vi "test_Configure Response_Variable Names Error.vi"(8 "error in (no error)":errorcluster, 11 "TestCase in":refnum<class "Instrument Addon Scripting API Messages Unit Tests.lvclass">) -> (0 "error out":errorcluster, 3 "TestCase out":refnum<class "Instrument Addon Scripting API Messages Unit Tests.lvclass">)   [LabVIEW 2019, in "Instrument Addon Scripting API Messages Unit Tests.lvclass"]
uses:
  Instrument Addon Scripting API Messages Unit Tests.lvclass
  APIs/Scripting API/TypeDefs/Wait Response Settings.ctl
  APIs/Scripting API/TypeDefs/Linked Channel.ctl
  <vilib>/NI VeriStand/Custom Device API/Custom Device Item Ref.ctl
  Instrument Addon Scripting API Messages Unit Tests.lvclass/Instrument Addon Scripting API Messages Unit Tests.ctl
  Addon/Addon Shared/SubVIs/Constants.vi
  <vilib>/NI/NI VeriStand Advanced SysDef API/_SubVIs/SysDef.Search.GUID.vi
  APIs/Scripting API/Messages/Configure Response - Wait (sec).vi
  <vilib>/addons/_JKI Toolkits/VI Tester/TestCase.llb/TestCase.lvclass
  Instrument Addon Scripting API Test Assets/Instrument Addon Scripting API Test Assets.lvclass
  APIs/Scripting API/Instrument Addon Scripting API.lvlib
  <vilib>/NI VeriStand/Custom Device API/Custom Device API.lvlib
  <vilib>/NI/NI VeriStand Advanced SysDef API/SysDef API/Advanced System Definition.lvlib
  Addon/Addon Shared/Instrument Addon Shared.lvlib
  C:/Program Files (x86)/National Instruments/LabVIEW 2019/vi.lib/addons/_JKI Toolkits/VI Tester/TestCase.llb/TestCase.lvclass
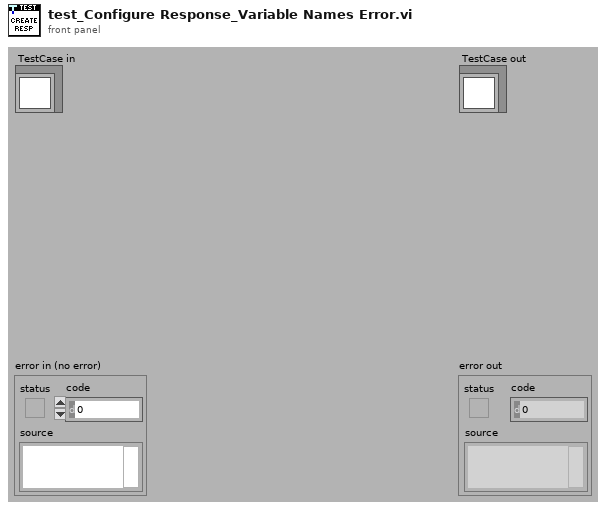
[diagram p1: front panel]
types:
  T1 = typedef "Instrument Addon Scripting API.lvlib/Wait Response Settings.ctl" = cluster{"Response Format":string, "Linked Channels":T2[], "Wait value (sec)":dbl, "Use Wait Channel":bool, "Channel Refnum":T3}
  T2 = typedef "Instrument Addon Scripting API.lvlib/Linked Channel.ctl" = cluster{"Variable Name":string, "Channel Refnum":T3}
  T3 = typedef "Custom Device API.lvlib/Custom Device Item Ref.ctl" = u64
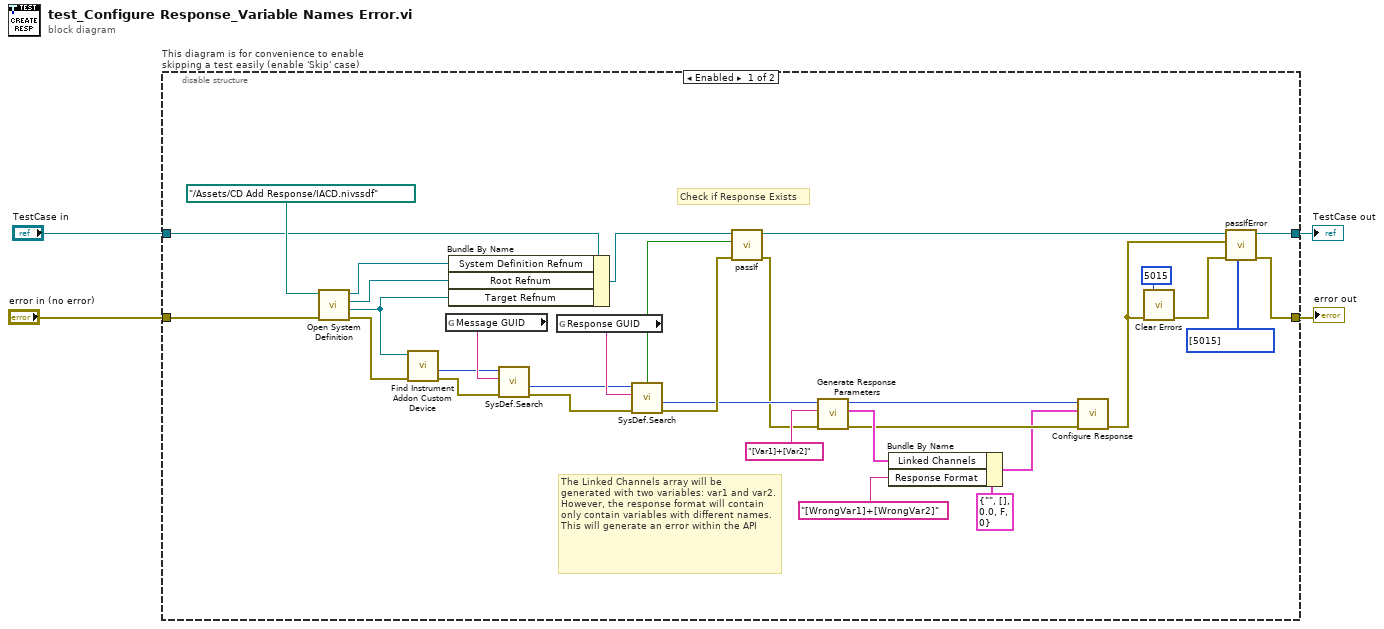
[diagram p0: block diagram]
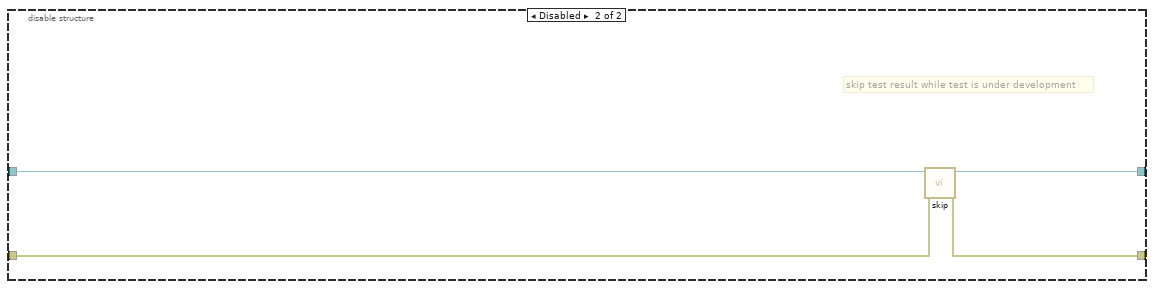
[diagram p2: hidden frame]
diagram:
  n1 = disable-structure "This diagram is for convenience to enable skipping a test easily (enable 'Skip' case)" shown="Enabled" {
    disable-tunnel: "TestCase in" -> [w10 w40]
    disable-tunnel: [w29 w38] -> w1
    disable-tunnel: [w28 w39] -> w3
    disable-tunnel: "error in (no error)" -> [w35 w37]
    frame Enabled {
      # "The Linked Channels array will be \ngenerated with two variables: var1 and var2. However, the response format will contain only contain variables with different names. This will generate an error within the API"
      # "Check if Response Exists"
      n2 = call "Open System Definition.vi"("error in (no error)"=w35, "System Definition File"=path "../Assets/CD Add Response/IACD.nivssdf" ("SDF file")) -> ("error out"=w34:errorcluster, "Target Refnum"=w8:refnum<k24>, "Root Refnum"=w7:refnum<k24>, "System Definition Refnum"=w6:refnum<k24>)  [unwired: 6 in]
      n3 = call "Find Instrument Addon Custom Device.vi"("error in"=w34, "target in"=w8) -> ("error out"=w24:errorcluster, "NodeID"=w23:u64)  [unwired: 7 in, 1 out]
      n4 = global read "Constants.vi" "Message GUID"() -> (w25:string)
      n5 = Bundle By Name(cluster=w10, "System Definition Refnum"=w6, "Root Refnum"=w7, "Target Refnum"=w8) -> (w9:refnum<class "Instrument Addon Scripting API Messages Unit Tests.lvclass">)
      n6 = call-poly <vilib>:"SysDef.Search.vi"("error in (no error)"=w24, "GUID"=w25, "nodeID"=w23) -> ("error out"=w21:errorcluster, "Value out"=w22:u64)  [unwired: 5 in, 2 out]
      n7 = global read "Constants.vi" "Response GUID"() -> (w33:string)
      n8 = call-poly <vilib>:"SysDef.Search.vi"("error in (no error)"=w21, "GUID"=w33, "nodeID"=w22) -> ("error out"=w20:errorcluster, "Value out"=w19:u64, "Found?"=w32:bool)  [unwired: 5 in, 1 out]
      n9 = call-dynamic "passIf.vi"("error in (no error)"=w20, "pass"=w32, "TestCase in"=w9) -> ("error out"=w17:errorcluster, "TestCase out"=w30:refnum<class "Instrument Addon Scripting API Messages Unit Tests.lvclass">)  [unwired: 7 in]
      n10 = call "Generate Response Parameters.vi"("Error In"=w17, "Response String"="[Var1]+[Var2]" ("Response Format"), "Response Channel in"=w19) -> ("Error Out"=w14:errorcluster, "Linked Channels"=w16:T2[], "Response Channel out"=w5:T3)  [unwired: 5 in, 1 out]
      n11 = Bundle By Name(cluster=T1 {"Response Format"="", "Linked Channels"=[], "Wait value (sec)"=0.0, "Use Wait Channel"=FALSE, "Channel Refnum"=0} ("Settings"), "Linked Channels"=w16, "Response Format"="[WrongVar1]+[WrongVar2]") -> (w13:T1)
      n12 = call-poly "Configure Response.vi"("error in (no error)"=w14, "settings"=w13, "reponse refnum in"=w5) -> ("error out"=w11:errorcluster)  [unwired: 7 in, 1 out]
      n13 = call <vilib>:"Clear Errors.vi"("error in (no error)"=w11, "specific error code to clear (0: all)"=5015) -> ("error out"=w26:errorcluster)  [unwired: 4 in, 1 out]
      n14 = call-dynamic "passIfError.vi"("passing error codes (default = any error code)"=i32[] [5015], "error in (no error)"=w26, "error"=w11, "TestCase in"=w30) -> ("error out"=w28:errorcluster, "TestCase out"=w29:refnum<class "Instrument Addon Scripting API Messages Unit Tests.lvclass">)  [unwired: 6 in]
    }
    frame Disabled {
      # "skip test result while test is under development"
      n15 = call <vilib>:"skip.vi"("error in (no error)"=w37, "TestCase in"=w40) -> ("error out"=w39:errorcluster, "TestCase out"=w38:refnum<class "Instrument Addon Scripting API Messages Unit Tests.lvclass">)  [unwired: 8 in]
    }
  }
  "error out" <- w3
  "TestCase out" <- w1
